vi "Get Project LV Version.vi"() -> ()   [LabVIEW 2012]
uses:
  msvcrt.dll
panel:
  out "error out":errorcluster
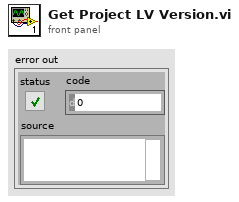
[diagram p1: front panel]
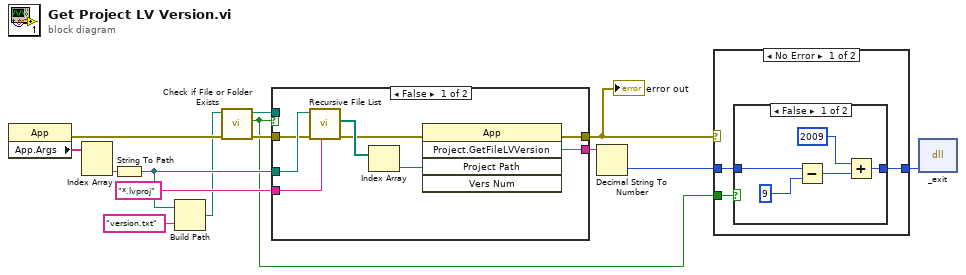
[diagram p0: block diagram]
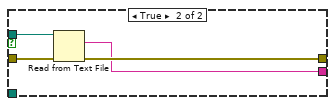
[diagram p2: hidden frame]
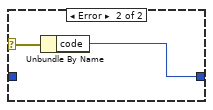
[diagram p4: hidden frame]
diagram:
  n1 = property class="App"() -> (error out=w7:errorcluster, "App.Args"=w12:string[])  [unwired: 2 in, 1 out]
  n2 = Index Array(array=w12) -> (element #2=w11:string)  [unwired: 2 in, 1 out]
  n3 = String To Path(string=w11) -> (path=w9:path)
  n4 = Build Path(base path=w9, name or relative path="version.txt") -> (appended path=w6:path)
  n5 = call <vilib>:"Check if File or Folder Exists.vi"("error in (no error)"=w7, "path"=w6) -> ("error out"=w5:errorcluster, "file or folder exists?"=w1:bool, "dup path"=w4:path)  [unwired: 7 in]
  n6 = case shown="False" w1 {
    tunnel: "*.lvproj" ("pattern") -> [w22 _]
    tunnel: [w16 w24] -> w13
    tunnel: w9 -> [w20 _]
    tunnel: w5 -> [w19 w26]
    tunnel: w4 -> [_ w25]
    tunnel: [w15 w23] -> w3
    frame False {
      n7 = call <vilib>:"Recursive File List.vi"("pattern"=w22, "error in (no error)"=w19, "Folder Path"=w20) -> ("error out"=w17:errorcluster, "All Files in Dir"=w21:path[])  [unwired: 4 in, 3 out]
      n8 = Index Array(array=w21) -> (element=w18:path)  [unwired: 1 in]
      n9 = invoke class="App" method="Project.GetFileLVVersion"(error in=w17, "Project Path"=w18) -> (error out=w16:errorcluster, "Project.GetFileLVVersion"=w15:string)  [unwired: 3 in, 3 out]
    }
    frame True {
      n10 = Read from Text File(file (use dialog)=w25, error in=w26) -> (text=w23:string, error out=w24:errorcluster)  [unwired: 2 in, 2 out]
    }
  }
  "error out" <- w13
  n11 = Decimal String To Number(string=w3) -> (number=w2:i32)  [unwired: 2 in, 1 out]
  n12 = case shown="No Error" w13 {
    selector: w13 -> [_ w37]
    tunnel: [w29 w36] -> w14
    tunnel: w2 -> [w28 _]
    tunnel: w1 -> [w27 _]
    frame No Error {
      n13 = case shown="False" w27 {
        tunnel: w28 -> [w34 w35]
        tunnel: [w30 w35] -> w29
        frame False {
          n14 = Subtract(x=w34, y=9) -> (x-y=w32:i32)
          n15 = Add(x=2009, y=w32) -> (x+y=w30:i32)
        }
        frame True {
        }
      }
    }
    frame Error {
      n16 = Unbundle By Name(w37) -> ("code"=w36:i32)
    }
  }
  n17 = dll-call lib="msvcrt.dll" fn="_exit"("status"=w14) -> ()  [unwired: 5 in, 2 out]
